vi "Dummy Scan.vi"(8 "error in (no error)":errorcluster, 11 "Dummy Scan in":refnum<class "Dummy Scan.lvclass">) -> (0 "error out":errorcluster, 3 "Dummy Scan out":refnum<class "Dummy Scan.lvclass">)   [LabVIEW 2012, in "Dummy Scan.lvclass"]
uses:
  Dummy Scan.lvclass
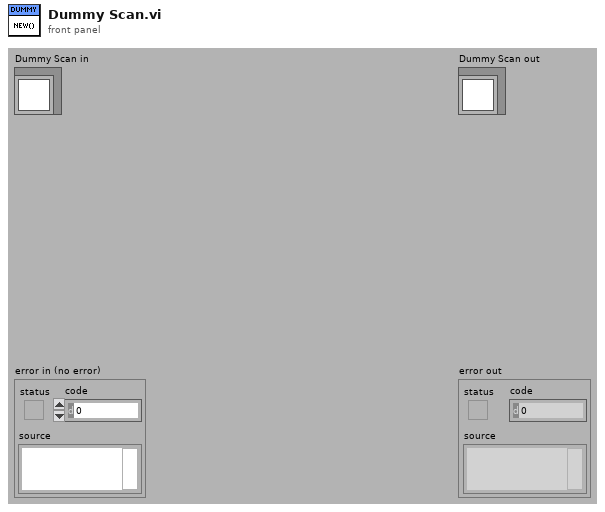
[diagram p1: front panel]
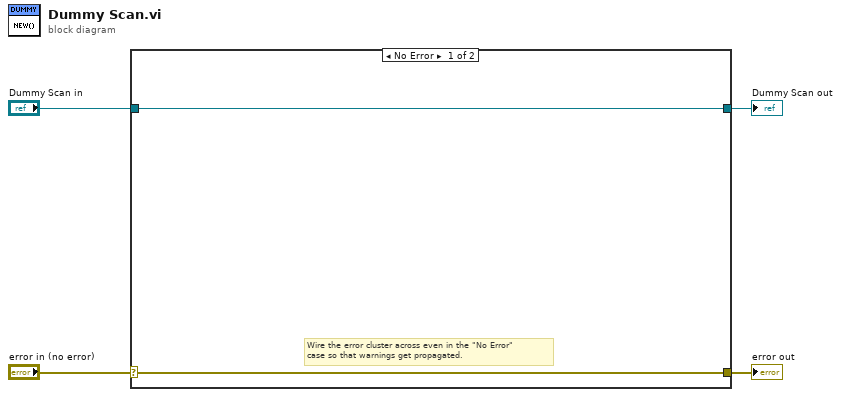
[diagram p0: block diagram]
diagram:
  n1 = case shown="No Error" "error in (no error)" {
    selector: "error in (no error)" -> [w5 w8]
    tunnel: [w5 w8] -> w3
    tunnel: [w6 w7] -> w1
    tunnel: "Dummy Scan in" -> [w6 w7]
    frame No Error {
      # "Wire the error cluster across even in the \"No Error\"\ncase so that warnings get propagated."
    }
    frame Error {
    }
  }
  "error out" <- w3
  "Dummy Scan out" <- w1
